vi "Pulse Generator.vi"() -> ()   [LabVIEW 2020]
uses:
  <vilib>/DAQmx/create/channels.llb/DAQmx Create Channel (CO-Pulse Generation-Time).vi
  <vilib>/DAQmx/configure/timing.llb/DAQmx Timing (Implicit).vi
  <vilib>/DAQmx/configure/trigger.llb/DAQmx Start Trigger (Digital Edge).vi
  <resource>/objmgr/daqmx.rc
panel:
  in  "Output Pulse":tag
  in  "stop":bool
  in  "Trigger":tag
  in  "Low Time":dbl=0.0001
  in  "High Time":dbl=0.00025
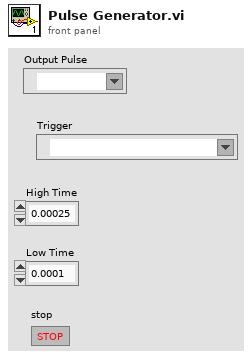
[diagram p1: front panel]
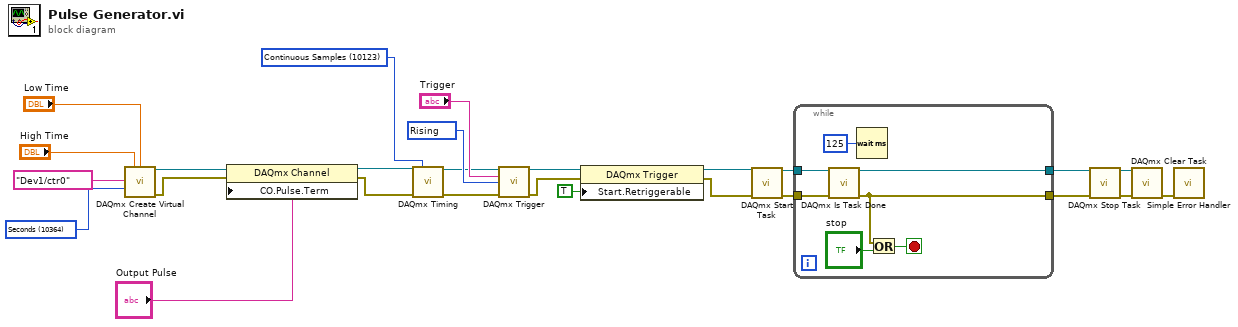
[diagram p0: block diagram]
diagram:
  w16 = 10123 items=["Finite Samples"=10178, "Continuous Samples"=10123, "Hardware Timed Single Point"=12522] ("sample mode")
  w19 = 10364 items=["Seconds"=10364] ("units")
  w25 = 10280 items=["Rising"=10280, "Falling"=10171] ("edge")
  n1 = call-poly <vilib>:"DAQmx Create Virtual Channel.vi"("high time"="High Time", "low time"="Low Time", "counter"=tag "Dev1/ctr0", "units"=w19) -> ("task out"=w6:refnum<k21>, "error out"=w5:errorcluster)  [unwired: 10 in]
  n2 = property class="DAQmx Channel"(reference=w6, error in=w5, "CO.Pulse.Term"="Output Pulse") -> (reference out=w4:refnum<k21>, error out=w3:errorcluster)
  n3 = call-poly <vilib>:"DAQmx Timing.vi"("task/channels in"=w4, "sample mode"=w16, "error in"=w3) -> ("task out"=w17:refnum<k21>, "error out"=w18:errorcluster)  [unwired: 11 in]
  n4 = call-poly <vilib>:"DAQmx Trigger.vi"("task/channels in"=w17, "source"="Trigger", "edge"=w25, "error in"=w18) -> ("task out"=w11:refnum<k21>, "error out"=w10:errorcluster)  [unwired: 10 in]
  n5 = property class="DAQmx Trigger"(reference=w11, error in=w10, "Start.Retriggerable"=TRUE) -> (reference out=w9:refnum<k21>, error out=w8:errorcluster)
  n6 = call <vilib>:"DAQmx Start Task.vi"("task/channels in"=w9, "error in"=w8) -> ("task out"=w15:refnum<k21>, "error out"=w14:errorcluster)  [unwired: 12 in]
  n7 = while {
    tunnel: w15 -> [w33]
    tunnel: w14 -> [w32]
    tunnel: [w31] -> w13
    tunnel: [w30] -> w12
    stop <- w28 stop-if-true
    n8 = call <vilib>:"DAQmx Is Task Done.vi"("task/channels in"=w33, "error in"=w32) -> ("task out"=w31:refnum<k21>, "error out"=w30:errorcluster)  [unwired: 11 in, 1 out]
    n9 = Wait (ms)(milliseconds to wait=u32 125) -> ()  [unwired: 1 out]
    n10 = Or(x=w30, y="stop") -> (x .or. y?=w28:bool)
  }
  n11 = call <vilib>:"DAQmx Stop Task.vi"("task/channels in"=w13, "error in"=w12) -> ("task out"=w23:refnum<k21>, "error out"=w24:errorcluster)  [unwired: 12 in]
  n12 = call <vilib>:"DAQmx Clear Task.vi"("task in"=w23, "error in"=w24) -> ("error out"=w22:errorcluster)  [unwired: 13 in]
  n13 = call <vilib>:"Simple Error Handler.vi"("error in (no error)"=w22) -> ()  [unwired: 4 in, 5 out]
